vi "Quality_Details.vi"() -> ()   [LabVIEW 2020]
doc: "Fonction :\n\nCe modèle peut être intégré très facilement à un subpannel à l'aide des fonctions de la palette Code Template >> Dynamic VI and Subpanel de la VIBOX"
uses:
  System.Windows.Forms
  <vilib>/DataGrid for LabVIEW/source/GridColumn/ColumnDefinition.ctl
  <vilib>/DataGrid for LabVIEW/source/GridColumn/ColumnType.ctl
  <vilib>/Utility/NIReport.llb/Report Type.ctl
  <vilib>/Utility/NIReport.llb/Append Text Table to Report (wrap).vi
  <vilib>/DataGrid for LabVIEW/source/DataTable/DataTable.lvclass
  <vilib>/DataGrid for LabVIEW/source/DataGridView/DataGridView.lvclass
  C:/Program Files (x86)/National Instruments/LabVIEW 2020/examples/DataGrid for LabVIEW/DataGrid.lvlib
  <vilib>/DataGrid for LabVIEW/source/GridColumn/GridColumn.lvclass
  <vilib>/DataGrid for LabVIEW/source/Events/CellClick/CellClick.lvclass
  <vilib>/Utility/NIReport.llb/NI_report.lvclass
  <vilib>/Utility/NIReport.llb/NI_ReportGenerationCore.lvlib
panel:
  out "data":string[][](array[string])
  out "Report<user event>":refnum<user-event>
  out "Stop":bool
  out "column":i32
  out "row":i32
  in  "DataGrid":refnum<k24>(container)
  out "Stop<user event>":refnum<user-event>
  in  "查看报表":bool
  in  "导出":bool
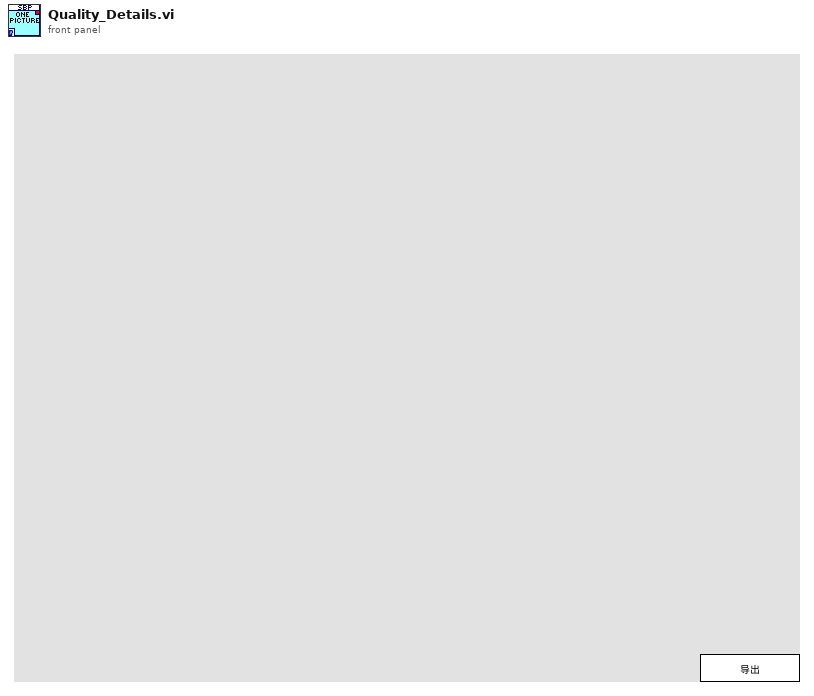
[diagram p1: front panel]
types:
  T1 = typedef "DataGrid.lvlib/GridColumn.lvclass/ColumnDefinition.ctl" = cluster{"name":string, "caption":string, "datatype":T2, "Params":string, "AutoSizeMode":i32, "FillWeight":sgl, "MinWidth":u32, "tooltip":string}
  T2 = typedef "DataGrid.lvlib/GridColumn.lvclass/ColumnType.ctl" = enum16{"string", "image", "check", "numeric", "timestamp", "button", "combo", "link"}
  T3 = typedef "NI_ReportGenerationCore.lvlib/Report Type.ctl" = enum16{"HTML", "Word", "Excel"}
  T4 = enum16{"maximized", "minimized", "normal", "no change"}
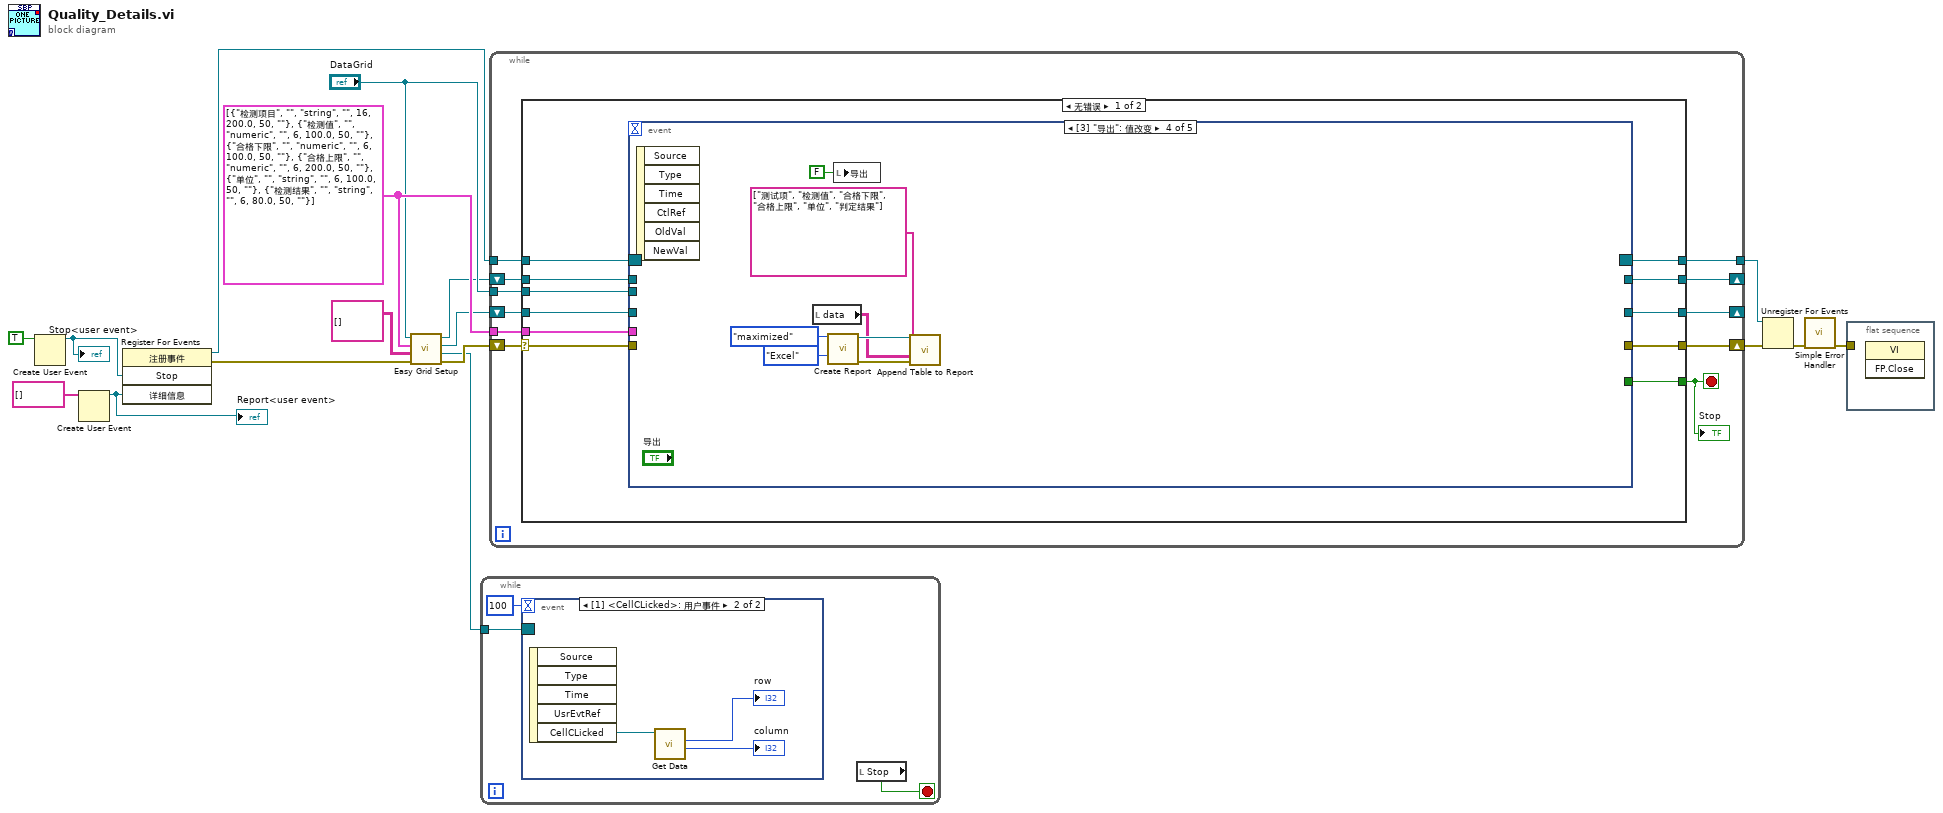
[diagram p0: block diagram]
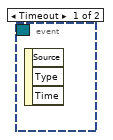
[diagram p2: hidden frame]
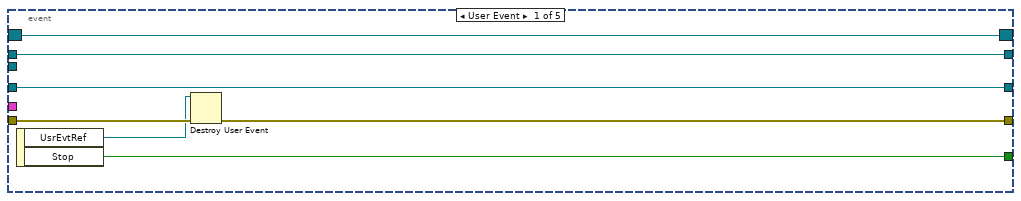
[diagram p3: hidden frame]
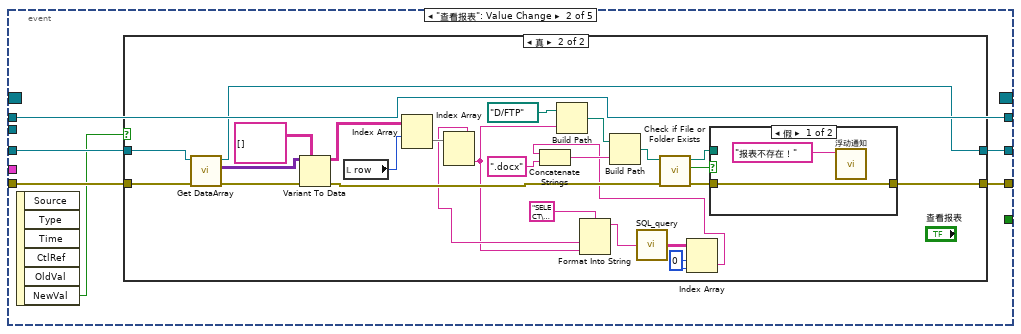
[diagram p4: hidden frame]
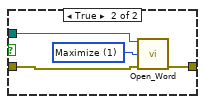
[diagram p6: hidden frame]
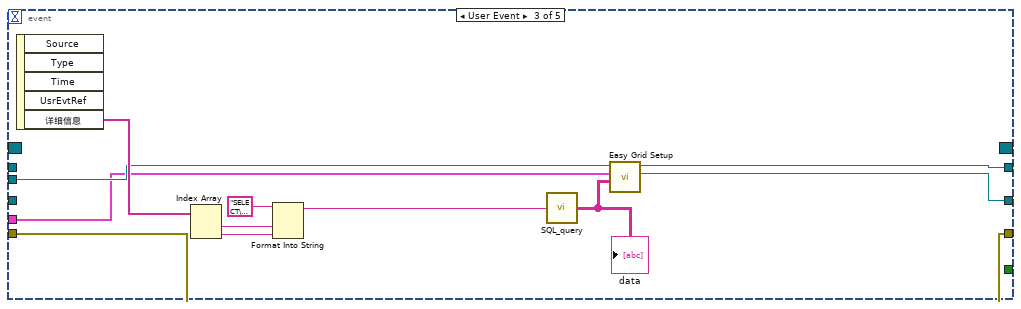
[diagram p7: hidden frame]
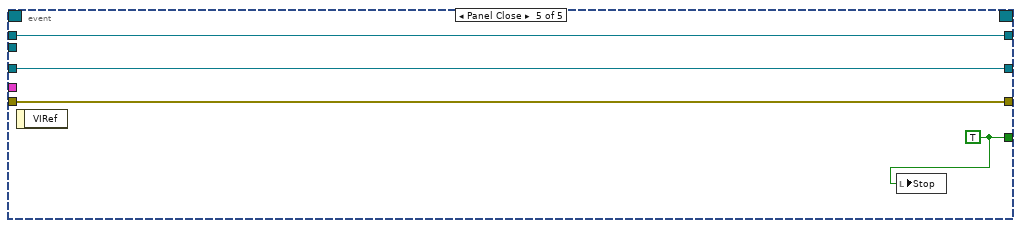
[diagram p8: hidden frame]
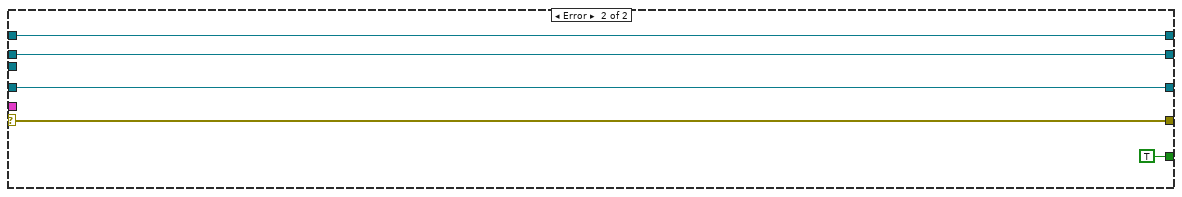
[diagram p9: hidden frame]
diagram:
  w8 = T1[] [{"name"="检测项目", "caption"="", "datatype"=enum."string", "Params"="", "AutoSizeMode"=16, "FillWeight"=200.0, "MinWidth"=50, "tooltip"=""}, {"name"="检测值", "caption"="", "datatype"=enum."numeric", "Params"="", "AutoSizeMode"=6, "FillWeight"=100.0, "MinWidth"=50, "tooltip"=""}, {"name"="合格下限", "caption"="", "datatype"=enum."numeric", "Params"="", "AutoSizeMode"=6, "FillWeight"=100.0, "MinWidth"=50, "tooltip"=""}, {"name"="合格上限", "caption"="", "datatype"=enum."numeric", "Params"="", "AutoSizeMode"=6, "FillWeight"=200.0, "MinWidth"=50, "tooltip"=""}, {"name"="单位", "caption"="", "datatype"=enum."string", "Params"="", "AutoSizeMode"=6, "FillWeight"=100.0, "MinWidth"=50, "tooltip"=""}, {"name"="检测结果", "caption"="", "datatype"=enum."string", "Params"="", "AutoSizeMode"=6, "FillWeight"=80.0, "MinWidth"=50, "tooltip"=""}] ("ColumnSetup")
  n1 = Create User Event(user event datatype=TRUE ("Stop")) -> (user event=w15:refnum<user-event>)  [unwired: 1 in, 1 out]
  "Stop<user event>" <- w15
  n2 = Create User Event(user event datatype=string[] [] ("详细信息")) -> (user event=w9:refnum<user-event>)  [unwired: 1 in, 1 out]
  "Report<user event>" <- w9
  n3 = register-events(w15, w9) -> (reference out=w14:refnum<event-registration>, error out=w4:errorcluster)  [unwired: 2 in]
  n4 = call <vilib>:"Easy Grid Setup.vi"("error in"=w4, "DataSource Data"=string[][] [], "ColumnSetup"=w8, "DataGridView"="DataGrid") -> ("error out"=w3:errorcluster, "registeredEvents"=w1:refnum<event-registration>, "DataTable out"=w5:refnum<class "DataTable.lvclass">, "DataGrid out"=w6:refnum<class "DataGridView.lvclass">)  [unwired: 4 in]
  n5 = while {
    tunnel: w1 -> [w20]
    stop <- w19 stop-if-true
    n6 = event shown="[1] <CellCLicked>: 用户事件" {
      selector: w20 -> [_ _]
      dyn-events: _ -> [_ _]
      timeout: 100 -> [_ _]
      event Timeout {
        n7 = event-data() -> ()  [unwired: 1 in, 3 out]
      }
      event User Event {
        n8 = event-data() -> ("CellCLicked"=w23:refnum<class "Abstract EVENT.lvclass">)  [unwired: 1 in, 4 out]
        n9 = call <vilib>:"Get Data.vi"("DataGrid.lvlib:Abstract EVENT.lvclass"=w23) -> ("column"=→"column":i32, "row"=→"row":i32)  [unwired: 8 in, 1 out]
      }
    }
    n10 = local read "Stop"() -> (w19:bool)
  }
  n11 = while {
    tunnel: w14 -> [w32]
    tunnel: [w31] -> w17
    shift-right: [w33] -> w13
    shift-left: w3 -> [w34]
    tunnel: "DataGrid" -> [w30]
    tunnel: w8 -> [w29]
    shift-right: [w28] -> _
    shift-left: w6 -> [w26]
    shift-right: [w27] -> _
    shift-left: w5 -> [w25]
    stop <- w24 stop-if-true
    n12 = case shown="无错误" w34 {
      selector: w34 -> [w42 w118]
      tunnel: [w41 w118] -> w33
      tunnel: [w43 TRUE] -> w24
      tunnel: w32 -> [w44 w117]
      tunnel: [w45 w117] -> w31
      tunnel: w30 -> [w40 _]
      tunnel: w29 -> [w39 _]
      tunnel: [w38 w116] -> w28
      tunnel: [w37 w115] -> w27
      tunnel: w26 -> [w36 w116]
      tunnel: w25 -> [w35 w115]
      frame No Error {
        n13 = event shown="[3] \"导出\": 值改变" {
          selector: w44 -> [w52 _ _ _ _]
          dyn-events: [w52 _ _ _ _] -> w45
          timeout: _ -> [_ _ _ _ _]
          tunnel: [w49 _ _ _ w113] -> w43
          tunnel: w42 -> [w51 w56 w97 _ w114]
          tunnel: [w48 w55 w97 _ w114] -> w41
          tunnel: w40 -> [_ _ w102 _ _]
          tunnel: w39 -> [_ _ w99 _ _]
          tunnel: [w47 w57 w101 _ w111] -> w38
          tunnel: [w46 w54 w100 _ w112] -> w37
          tunnel: w36 -> [w47 w57 _ _ w111]
          tunnel: w35 -> [w46 w58 _ _ w112]
          event User Event {
            n14 = event-data() -> ("UsrEvtRef"=w50:refnum<user-event>, "Stop"=w49:bool)  [unwired: 1 out]
            n15 = Destroy User Event(user event=w50, error in=w51) -> (error out=w48:errorcluster)
          }
          event "查看报表": Value Change {
            n16 = event-data() -> ("NewVal"=w53:bool)  [unwired: 6 out]
            n17 = case shown="真" w53 {
              tunnel: w58 -> [w60 w81]
              tunnel: w56 -> [w59 w73]
              tunnel: [w59 w69] -> w55
              tunnel: [w60 w68] -> w54
              frame False {
              }
              frame True {
                w62 = 0 ("索引 (行)")
                n18 = call <vilib>:"Get DataArray.vi"("error in (no error)"=w73, "DataTable in"=w81) -> ("error out"=w72:errorcluster, "Array"=w86:variant[][], "DataTable out"=w68:refnum<class "DataTable.lvclass">)  [unwired: 7 in]
                n19 = Variant To Data(error in=w72, type=string[][] [], Variant=w86) -> (data=w84:string[][], error out=w71:errorcluster)
                n20 = local read "row"() -> (w83:i32)
                n21 = Index Array(array=w84, index (row)=w83) -> (element=w82:string[])  [unwired: 1 in]
                n22 = Index Array(array=w82) -> (element #1=w66:string, element #2=w64:string)  [unwired: 2 in]
                n23 = Build Path(base path=path "D:/FTP" ("基路径"), name or relative path=w64) -> (appended path=w79:path)
                n24 = Format Into String(format string="SELECT\ndbo.[产品质量2].[工位追溯码]\n\nFROM\ndbo.[产品质量2]\nWHERE\ndbo.[产品质量2].[总成追溯码] = N'%s' AND\ndbo.[产品质量2].[设备编号] = N'%s'\nGROUP BY\ndbo.[产品质量2].[工位追溯码]\n", w66, w64) -> (resulting string=w65:string)  [unwired: 2 in, 1 out]
                n25 = call "SQL_query.vi"("SQL query"=w65) -> ("data"=w63:string[][])  [unwired: 3 in, 1 out]
                n26 = Index Array(array=w63, index (row)=w62, index (col)=w62) -> (element=w61:string)
                n27 = Concatenate Strings(w61, ".docx" ("字符串")) -> (w77:string)
                n28 = Build Path(base path=w79, name or relative path=w77) -> (appended path=w76:path)
                n29 = call <vilib>:"Check if File or Folder Exists.vi"("error in (no error)"=w71, "path"=w76) -> ("error out"=w70:errorcluster, "file or folder exists?"=w75:bool, "dup path"=w74:path)  [unwired: 7 in]
                n30 = case shown="假" w75 {
                  tunnel: w74 -> [_ w92]
                  tunnel: w70 -> [w88 w90]
                  tunnel: [w88 w89] -> w69
                  frame False {
                    n31 = call "浮动通知.vi"("通知内容"="报表不存在！" ("消息")) -> ()  [unwired: 11 in]
                  }
                  frame True {
                    w91 = 1 items=["Normal", "Maximize", "Minimize"] ("cpubbs_WindowState")
                    n32 = call "Open_Word.vi"("File Path"=w92, "cpubbs_WindowState"=w91, "错误输入（无错误）"=w90) -> ("错误输出"=w89:errorcluster)  [unwired: 12 in]
                  }
                }
              }
            }
          }
          event User Event {
            n33 = event-data() -> ("详细信息"=w103:string[])  [unwired: 5 out]
            n34 = Index Array(array=w103) -> (element #1=w96:string, element #2=w93:string)  [unwired: 2 in]
            n35 = Format Into String(format string="SELECT\ndbo.Test.TEST_NAME,\ndbo.Test.TEST_VALUE,\ndbo.Test.TEST_VALUE_MIN,\ndbo.Test.TEST_VALUE_MAX,\ndbo.Test.TEST_VALUE_UNIT,\ndbo.Test.TEST_VALUE_RESULT\n\nFROM\ndbo.Test\nINNER JOIN dbo.Device ON dbo.Test.DEVICE_ID = dbo.Device.DEVICE_ID\nINNER JOIN dbo.Code ON dbo.Test.CODE_ID = dbo.Code.CODE_ID\nWHERE\ndbo.Code.CODE_ID = '%s' AND\ndbo.Device.DEVICE_NAME = '%s'\n\n", w96, w93) -> (resulting string=w94:string)  [unwired: 2 in, 1 out]
            n36 = call "SQL_query.vi"("SQL query"=w94) -> ("data"=w98:string[][])  [unwired: 3 in, 1 out]
            "data" <- w98
            n37 = call <vilib>:"Easy Grid Setup.vi"("DataSource Data"=w98, "ColumnSetup"=w99, "DataGridView"=w102) -> ("DataTable out"=w100:refnum<class "DataTable.lvclass">, "DataGrid out"=w101:refnum<class "DataGridView.lvclass">)  [unwired: 5 in, 2 out]
          }
          event "导出": Value Change {
            n38 = event-data() -> ()  [unwired: 7 out]
            n39 = local read "data"() -> (w105:string[][])
            n40 = call <vilib>:"Create Report.vi"("window state (normal)"=T4."maximized", "report type"=Report_Type."Excel") -> ("report out"=w107:refnum<class "NI_report.lvclass">, "error out"=w106:errorcluster)  [unwired: 12 in]
            n41 = local write "导出"(FALSE ("导出")) -> ()
            n42 = call-poly <vilib>:"Append Table to Report.vi"("report in"=w107, "column headers"=string[] ["测试项", "检测值", "合格下限", "合格上限", "单位", "判定结果"], "text data"=w105, "error in (no error)"=w106) -> ()  [unwired: 8 in, 4 out]
          }
          event Panel Close {
            w113 = TRUE ("Stop")
            n43 = event-data() -> ()  [unwired: 2 out]
            n44 = local write "Stop"(w113) -> ()
          }
        }
      }
      frame Error {
      }
    }
    "Stop" <- w24
  }
  n45 = Unregister For Events(event registration refnum=w17, error in=w13) -> (error out=w16:errorcluster)
  n46 = call <vilib>:"Simple Error Handler.vi"("error in (no error)"=w16) -> ("error out"=w11:errorcluster)  [unwired: 1 in, 7 out]
  n47 = flat-sequence {
    tunnel: w11 -> [_]
    frame #0 {
      n48 = invoke class="VI" method="FP.Close"() -> ()  [unwired: 3 in, 3 out]
    }
  }
